vi "AOTF-Trigger_pattern.vi"() -> ()   [LabVIEW 2011]
doc: "I. Description:\nThis example demonstrates how to generate a continuous digital pulse train from a Counter Output Channel started by an external digital trigger. The Frequency, Duty Cycle, and Idle State are all configurable. \n\nThis example shows how to configure the pulse in terms of Frequency/Duty Cycle, but can easily be modified to generate a pulse in terms of Time or Ticks.\n\nII. Instructions for Running:\n1. Select the Physical Channel which corresponds to the counter you want to output your signal to on the DAQ device.\n2. Enter the Frequency and Duty Cycle to define the pulse parameters. You can also change the Idle State to set the state the line will remain in after the generation is stopped. Additionally, you can set the Initial Delay (in seconds) which will delay the beginning of the pulse train from the start call; this is currently wired to 0.0 on the block diagram. \n3. Setup the Trigger Parameters. In this example the VI is expecting a Rising Edge Digital Trigger on PFI9. \n\nIII. Block Diagram Steps:\n1. Create a Counter Output channel to produce a Pulse in terms of Frequency. If the Idle State of the pulse is set to low the first transition of the generated signal is from low to high.\n2. Use the DAQmx Trigger VI to configure a trigger to start on a digital edge.\n2. Use the DAQmx Timing VI (Implicit) to configure the duration of the pulse generation.\n3. Call the Start VI to arm the counter and begin the pulse train generation.\n4. Loop continuously until the user presses the Stop button. Check for errors every 100 ms using the Is Task Done? VI\n5. Call the Clear Task VI to clear the Task.\n\nIV. I/O Connections Overview:\nThe counter will output the pulse train on the output terminal of the counter specified in the Physical Channel I/O control. \n\nIn this example the output will be sent to the default output terminal on ctr0.\n\nFor more information on the default counter input and output terminals for your device, open the NI-DAQmx Help, and refer to Counter Signal Connections found under the Device Considerations book in the table of contents."
uses:
  <vilib>/Utility/error.llb/DialogType.ctl
  <vilib>/DAQmx/create/channels.llb/DAQmx Create Channel (CO-Pulse Generation-Frequency).vi
  <vilib>/DAQmx/create/channels.llb/DAQmx Create Channel (DO-Digital Output).vi
  <vilib>/DAQmx/configure/timing.llb/DAQmx Timing (Implicit).vi
  Program Files (x86)/National Instruments/LabVIEW 2011/resource/objmgr/daqmx.rc
panel:
  in  "Duty Cycle":dbl=0.5 format="%0.2f"
  in  "Frequency":dbl=1.0 caption="Frequency (kHz)" format="%0.2f"
  in  "Stop":bool caption="stop"
  # "Channel Parameters"
  # "Trigger Parameters"
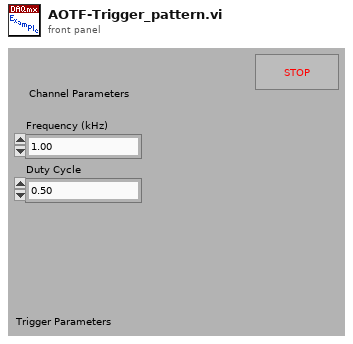
[diagram p1: front panel]
types:
  T1 = typedef "DialogType.ctl" = u16
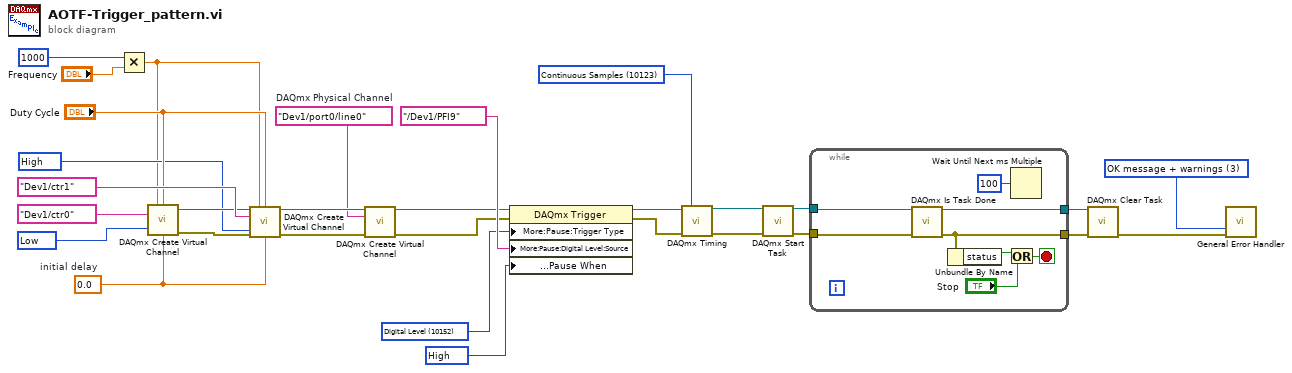
[diagram p0: block diagram]
diagram:
  w1 = tag "Dev1/port0/line0"  # DAQmx Physical Channel
  w7 = 10192 items=["High"=10192, "Low"=10214] ("Pause When")
  w6 = 10152 items=["Analog Level"=10101, "Analog Window"=10103, "Digital Level"=10152, "None"=10230] ("Pause.TrigType")
  w17 = 10214 items=["High"=10192, "Low"=10214] ("Idle State 2")
  w16 = 10192 items=["High"=10192, "Low"=10214] ("Idle State")
  w23 = T1 3 items=["no dialog", "OK message", "continue or stop message", "OK message + warnings", "continue/stop + warnings"] ("type of dialog (OK msg:1)")
  w19 = 0.0  # initial delay
  w26 = 10123 items=["Finite Samples"=10178, "Continuous Samples"=10123] ("sample mode")
  n1 = Multiply(x=1000, y="Frequency") -> (x*y=w15:dbl)
  n2 = call-poly <vilib>:"DAQmx Create Virtual Channel.vi"("frequency"=w15, "duty cycle"="Duty Cycle", "counter"=tag "Dev1/ctr0" ("Counter 2"), "idle state"=w17, "initial delay"=w19) -> ("task out"=w18:refnum<k21>, "error out"=w20:errorcluster)  [unwired: 9 in]
  n3 = call-poly <vilib>:"DAQmx Create Virtual Channel.vi"("task in"=w18, "frequency"=w15, "duty cycle"="Duty Cycle", "counter"=tag "Dev1/ctr1" ("Counter 1"), "error in"=w20, "idle state"=w16, "initial delay"=w19) -> ("task out"=w5:refnum<k21>, "error out"=w3:errorcluster)  [unwired: 7 in]
  n4 = call-poly <vilib>:"DAQmx Create Virtual Channel.vi"("task in"=w5, "lines"=w1, "error in"=w3) -> ("task out"=w4:refnum<k21>, "error out"=w2:errorcluster)  [unwired: 11 in]
  n5 = property class="DAQmx Trigger"(reference=w4, error in=w2, "More:Pause:Trigger Type"=w6, "More:Pause:Digital Level:Source"=tag "/Dev1/PFI9" ("Trigger Source"), "More:Pause:Digital Level:Pause When"=w7) -> (reference out=w9:refnum<k21>, error out=w10:errorcluster)
  n6 = call-poly <vilib>:"DAQmx Timing.vi"("task/channels in"=w9, "sample mode"=w26, "error in"=w10) -> ("task out"=w27:refnum<k21>, "error out"=w28:errorcluster)  [unwired: 11 in]
  n7 = call <vilib>:"DAQmx Start Task.vi"("task/channels in"=w27, "error in"=w28) -> ("task out"=w12:refnum<k21>, "error out"=w11:errorcluster)  [unwired: 12 in]
  n8 = while {
    tunnel: w11 -> [w37]
    tunnel: w12 -> [w38]
    tunnel: [w36] -> w29
    tunnel: [w35] -> w24
    stop <- w33 stop-if-true
    n9 = call <vilib>:"DAQmx Is Task Done.vi"("task/channels in"=w38, "error in"=w37) -> ("task out"=w36:refnum<k21>, "error out"=w35:errorcluster)  [unwired: 11 in, 1 out]
    n10 = Unbundle By Name(w35) -> ("status"=w32:bool)
    n11 = Or(x=w32, y="Stop") -> (x .or. y?=w33:bool)
    n12 = Wait Until Next ms Multiple(millisecond multiple=u32 100) -> ()  [unwired: 1 out]
  }
  n13 = call <vilib>:"DAQmx Clear Task.vi"("task in"=w29, "error in"=w24) -> ("error out"=w30:errorcluster)  [unwired: 13 in]
  n14 = call <vilib>:"General Error Handler.vi"("type of dialog (OK msg:1)"=w23, "error in (no error)"=w30) -> ()  [unwired: 9 in, 5 out]
